vi "Remove (Almost) Duplicates from 1D Array (DBL).vi"(6 "epsilon (machine)":dbl=2.220446049250313e-16, 11 "Input Array":dbl[](array[numeric])) -> (0 "indices of removed elements":i32[](array[numeric]), 3 "Output Array":dbl[](array[numeric]))   [LabVIEW 2019]
doc: "This polymorphic VI removes all duplicate elements in <B>Input Array</B> and outputs the result as <B>Output Array</B>. It also outputs the <B>indices of removed elements<B>."
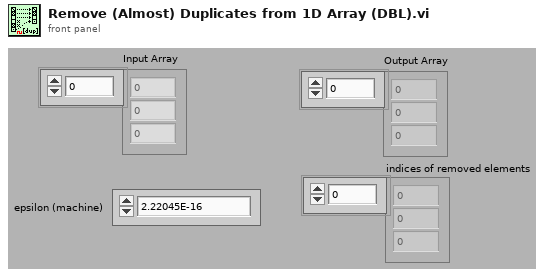
[diagram p1: front panel]
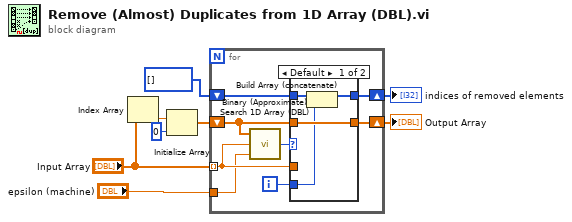
[diagram p0: block diagram]
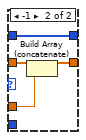
[diagram p2: hidden frame]
diagram:
  n1 = Index Array(array="Input Array") -> (element=w4:dbl)  [unwired: 1 in]
  n2 = Initialize Array(w4, 0 ("Dimension Size")) -> (w3:dbl[])
  n3 = for {
    tunnel: "Input Array" -> [w15] mode=indexing
    shift-right: [w14] -> w7
    shift-left: w3 -> [w13]
    shift-right: [w11] -> w5
    shift-left: i32[] [] -> [w10]
    tunnel: "epsilon (machine)" -> [w9]
    i -> [w12]
    n4 = call "Binary (Approximate) Search 1D Array (DBL).vi"("epsilon (machine)"=w9, "element"=w15, "1D array"=w13) -> ("index"=w16:i32)
    n5 = case shown="Default" w16 {
      tunnel: w15 -> [_ w24]
      tunnel: [w20 w22] -> w14
      tunnel: w13 -> [w20 w23]
      tunnel: w12 -> [w17 _]
      tunnel: [w18 w21] -> w11
      tunnel: w10 -> [w19 w21]
      frame Default {
        n6 = Build Array (concatenate)(w19, w17) -> (w18:i32[])
      }
      frame -1 {
        n7 = Build Array (concatenate)(w23, w24) -> (w22:dbl[])
      }
    }
  }
  "Output Array" <- w7
  "indices of removed elements" <- w5
